vi "SampleGetIDSingle.vi"() -> ()   [LabVIEW 2016]
panel:
  in  "DeviceKey In":string
  out "Identification":string
  out "error out":errorcluster
  out "DeviceKey Out":string
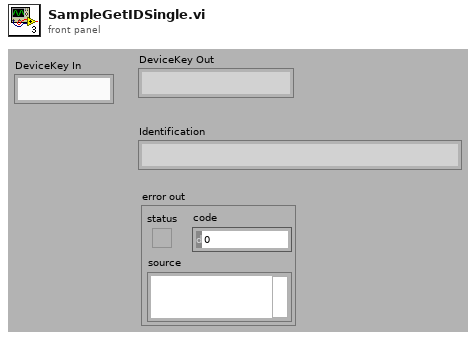
[diagram p1: front panel]
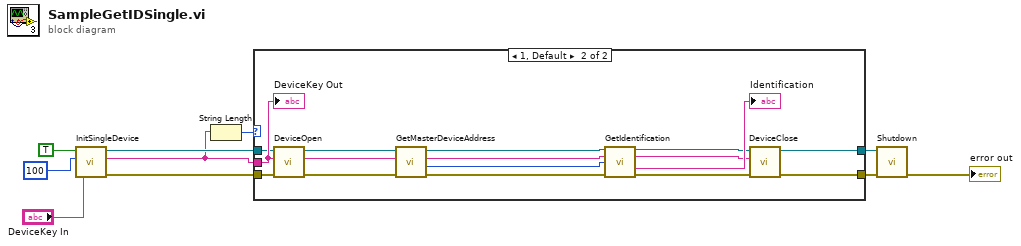
[diagram p0: block diagram]
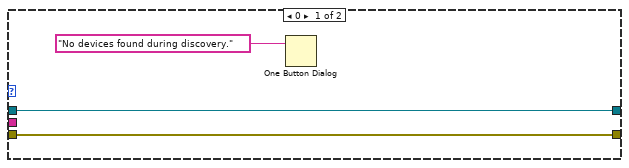
[diagram p2: hidden frame]
diagram:
  n1 = call "InitSingleDevice.vi"("deviceKey"="DeviceKey In", "msecDelayForDiscovery"=100, "logging"=TRUE) -> ("error out"=w3:errorcluster, "DeviceKey Out"=w2:string, "CmdLib Out"=w4:refnum<k24>)  [unwired: 2 in]
  n2 = String Length(string=w2) -> (length=w7:i32)
  n3 = case shown="1, Default" w7 {
    tunnel: [w13 w24] -> w6
    tunnel: [w12 w26] -> w5
    tunnel: w4 -> [w13 w15]
    tunnel: w3 -> [w12 w19]
    tunnel: w2 -> [_ w17]
    frame 0 {
      n4 = One Button Dialog(message="No devices found during discovery.") -> ()  [unwired: 1 in, 1 out]
    }
    frame 1, Default {
      n5 = call "DeviceOpen.vi"("error in (no error)"=w19, "DeviceKey In"=w17, "CmdLib In"=w15) -> ("error out"=w18:errorcluster, "DeviceKey Out"=w16:string, "CmdLib Out"=w14:refnum<k24>)  [unwired: 2 in]
      n6 = call "GetMasterDeviceAddress.vi"("error in (no error)"=w18, "DeviceKey In"=w16, "CmdLib In"=w14) -> ("error out"=w22:errorcluster, "Device Address"=w28:i32, "DeviceKey Out"=w20:string, "CmdLib Out"=w21:refnum<k24>)  [unwired: 1 in]
      n7 = call "GetIdentification.vi"("CmdLib In"=w21, "DeviceKey In"=w20, "Device Address In"=w28, "error in (no error)"=w22) -> ("CmdLib Out"=w25:refnum<k24>, "DeviceKey Out"=w23:string, "Identification"=→"Identification":string, "error out"=w27:errorcluster)  [unwired: 7 in, 1 out]
      n8 = call "DeviceClose.vi"("error in (no error)"=w27, "DeviceKey In"=w23, "CmdLib In"=w25) -> ("error out"=w26:errorcluster, "CmdLib Out"=w24:refnum<k24>)  [unwired: 2 in, 1 out]
      "DeviceKey Out" <- w17
    }
  }
  n9 = call "Shutdown.vi"("error in (no error)"=w5, "CmdLib In"=w6) -> ("error out"=→"error out":errorcluster)  [unwired: 4 in, 1 out]
